vi "Query Status Information.vi"(0 "VISA resource name":refnum<visa-resource-name>, 11 "error in (no error)":errorcluster) -> (4 "VISA resource name out":refnum<visa-resource-name>, 8 "Status Information":u8[](array[numeric]), 15 "error out":errorcluster)   [LabVIEW 2020, in "Yokogawa GX Series.lvlib"]
doc: "This VI gets the Status Information that is filtered.\nThe logical AND of the condition register and the filter becomes the status information."
uses:
  <instrlib>/Yokogawa GX Series/Yokogawa GX Series.lvlib
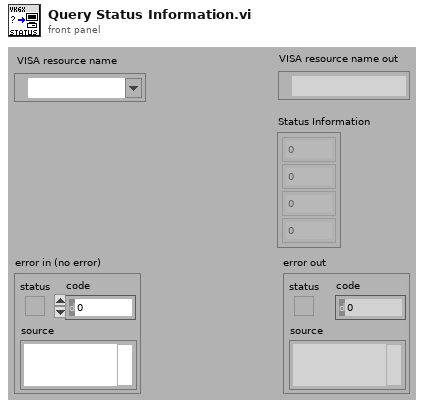
[diagram p1: front panel]
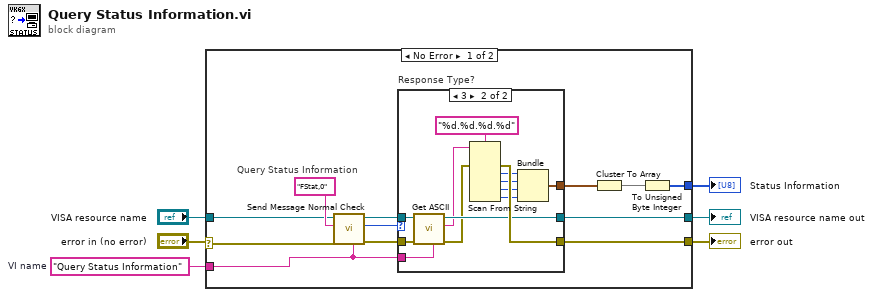
[diagram p0: block diagram]
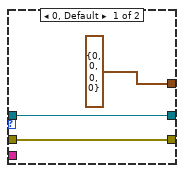
[diagram p2: hidden frame]
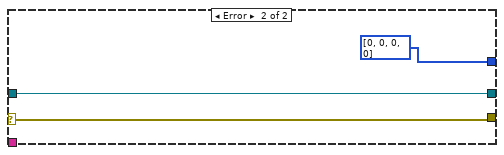
[diagram p3: hidden frame]
diagram:
  w4 = "Query Status Information"  # VI name
  n1 = case shown="No Error" "error in (no error)" {
    selector: "error in (no error)" -> [w7 w36]
    tunnel: [w18 w37] -> w6
    tunnel: [w17 w36] -> w5
    tunnel: w4 -> [w15 _]
    tunnel: [w10 u8[] [0, 0, 0, 0]] -> w3
    tunnel: "VISA resource name" -> [w8 w37]
    frame No Error {
      # "Query Status Information"
      n2 = call <instrlib>:"Send Message Normal Check.vi"("Source (\"\")"=w15, "error in (no error)"=w7, "Send Message (\"\")"="FStat,0", "VISA resource name"=w8) -> ("error out"=w12:errorcluster, "Response Type"=w13:i32, "VISA resource name out"=w14:refnum<visa-resource-name>)  [unwired: 1 in, 4 out]
      n3 = case "Response Type?" shown="3" w13 {
        tunnel: w14 -> [w21 w26]
        tunnel: w12 -> [w20 w27]
        tunnel: [w21 w25] -> w18
        tunnel: [w20 w34] -> w17
        tunnel: [cluster{i32, i32, i32, i32} {0, 0, 0, 0} ("クラスタ") w28] -> w16
        tunnel: w15 -> [_ w23]
        frame 0, Default {
        }
        frame 3 {
          n4 = call <instrlib>:"Get ASCII.vi"("Source (\"\")"=w23, "error in (no error)"=w27, "VISA resource name"=w26) -> ("error out"=w24:errorcluster, "ASCII Data"=w22:string, "VISA resource name out"=w25:refnum<visa-resource-name>)  [unwired: 6 out]
          n5 = Scan From String(format string="%d.%d.%d.%d", input string=w22, error in=w24) -> (error out=w34:errorcluster, output 1=w32:i32, output 2=w31:i32, output 3=w30:i32, output 4=w29:i32)  [unwired: 1 in, 6 out]
          n6 = Bundle(w32, w31, w30, w29) -> (w28:cluster{i32, i32, i32, i32})  [unwired: 1 out]
        }
      }
      n7 = Cluster To Array(cluster=w16) -> (array=w11:i32[])
      n8 = To Unsigned Byte Integer(number=w11) -> (unsigned 8bit integer=w10:u8[])
    }
    frame Error {
    }
  }
  "error out" <- w5
  "VISA resource name out" <- w6
  "Status Information" <- w3
